vi "FPGAPosition.vi"(2 "Calib Pt 1 (in)":sgl, 3 "Calib Pt 1 (amps)":sgl, 4 "Calib Pt 0 (in)":sgl, 5 "Calib Pt 0 (amps)":sgl) -> (0 "Block Position (in)":sgl, 1 "Mod3-9203/AI1":sgl)   [LabVIEW 2019]
uses:
  <vilib>/rvi/eio/common/nirviEmuTemplateMethod_errors.vi
  <vilib>/eio/EIONode/EIONode.xnode
  <vilib>/rvi/Analysis/measure/butterworth/XNode/niFpgaButterworthFilter.xnode
panel:
  # "READ Block Position"
  # "Banner Time of Flight Laser Distance Meter"
  # "(Amps)"
  # "Calibration Data"
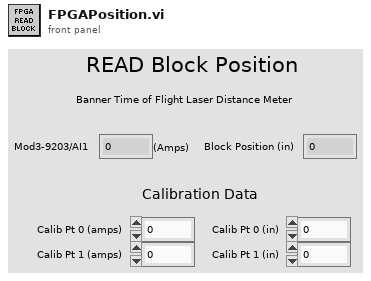
[diagram p1: front panel]
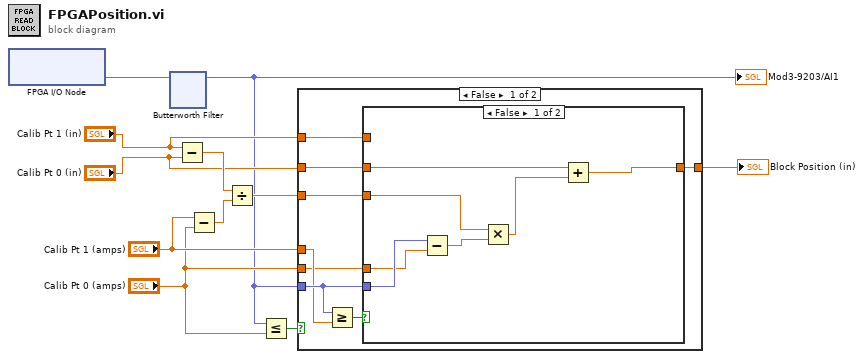
[diagram p0: block diagram]
diagram:
  n1 = xnode "FPGA I/O Node"() -> ("Mod3/AI1"=w1:fxp<+/-,21,-4>)  [unwired: 1 in, 1 out]
  n2 = xnode "Butterworth Filter"("input data"=w1) -> ("output data"=w2:fxp<+/-,25,0>)  [unwired: 2 in]
  "Mod3-9203/AI1" <- w2
  n3 = Subtract(x="Calib Pt 1 (in)", y="Calib Pt 0 (in)") -> (x-y=w9:sgl)
  n4 = Subtract(x="Calib Pt 1 (amps)", y="Calib Pt 0 (amps)") -> (x-y=w10:sgl)
  n5 = Divide(x=w9, y=w10) -> (x/y=w5:sgl)
  n6 = Less Or Equal?(x=w2, y="Calib Pt 0 (amps)") -> (x <= y?=w11:bool)
  n7 = case shown="False" w11 {
    tunnel: w2 -> [w15 _]
    tunnel: "Calib Pt 0 (in)" -> [w14 w28]
    tunnel: [w17 w28] -> w4
    tunnel: "Calib Pt 1 (amps)" -> [w13 _]
    tunnel: "Calib Pt 1 (in)" -> [w18 _]
    tunnel: w5 -> [w16 _]
    tunnel: "Calib Pt 0 (amps)" -> [w12 _]
    frame False {
      n8 = Greater Or Equal?(x=w15, y=w13) -> (x >= y?=w19:bool)
      n9 = case shown="False" w19 {
        tunnel: w18 -> [_ w27]
        tunnel: [w21 w27] -> w17
        tunnel: w16 -> [w24 _]
        tunnel: w15 -> [w26 _]
        tunnel: w14 -> [w23 _]
        tunnel: w12 -> [w20 _]
        frame False {
          n10 = Subtract(x=w26, y=w20) -> (x-y=w25:sgl)
          n11 = Multiply(x=w24, y=w25) -> (x*y=w22:sgl)
          n12 = Add(x=w23, y=w22) -> (x+y=w21:sgl)
        }
        frame True {
        }
      }
    }
    frame True {
    }
  }
  "Block Position (in)" <- w4
